vi "test_paylaod.vi"() -> ()   [LabVIEW 2021]
panel:
  out "output array":u8[](array[numeric])
  out "appended array":u8[](array[numeric])
  in  "Qac 1":dbl
  in  "Vdc 1":dbl
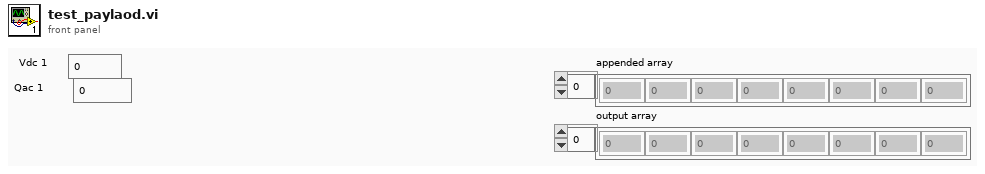
[diagram p1: front panel]
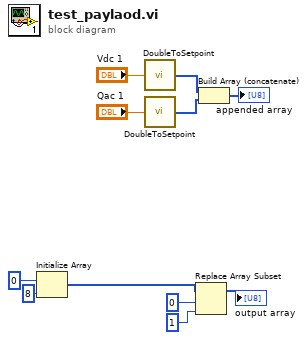
[diagram p0: block diagram]
diagram:
  n1 = Initialize Array(u8 0, 8 ("dimension size")) -> (w2:u8[])
  n2 = call "DoubleToSetpoint.vi"("Double"="Vdc 1") -> ("SP"=w9:u8[])
  n3 = call "DoubleToSetpoint.vi"("Double"="Qac 1") -> ("SP"=w8:u8[])
  n4 = Replace Array Subset(array=w2, new element=u8 1 ("new element/subarray"), index=0) -> (→"output array":u8[])
  n5 = Build Array (concatenate)(w9, w8) -> (→"appended array":u8[])
